vi "Controller 2 Functions.vi"(8 "AutoArmIn":u8, 10 "Controller in":string, 11 "Enabled?":enum16{"Disabled", "Enabled"}(ring)) -> (0 "AutoArm Out":u8)   [LabVIEW 2012, in "BlockParty4150.lvrbt"]
uses:
  BlockParty4150.lvrbt
  <vilib>/NXT/Hardware/Plugins/Tetrix DC Motor/TetrixDCMotorAddress.ctl
  <vilib>/NXT/Hardware/Plugins/Tetrix 180 deg Servo/Tetrix180ServoAddress.ctl
  <vilib>/FTC/FTC Calculate Drive Power - Tank.vi
  <vilib>/NXT/NXTIO Xnodes/NXTIONodeSubVIs/TETRIX IO Move DC Motors.vi
  <vilib>/NXT/NXTIO Xnodes/NXTIONodeSubVIs/TETRIX IO Move Servos.vi
  <vilib>/NXT/NXTIO Xnodes/AddressXNode/NXTIOAddress.xnode
  <vilib>/NXT/Subs/LVHSConnector.ctl
  <vilib>/NXT/NXTIO Xnodes/NXTIOXNode/NXTIO.xnode
  <vilib>/NXT/LegoClasses/BrickReference/BrickReference.lvclass
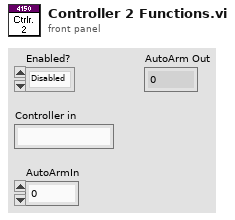
[diagram p1: front panel]
types:
  T1 = typedef "TetrixDCMotorAddress.ctl" = i32
  T2 = cluster{"TetrixDCMotor":T1, "TetrixDCMotor 2":T1}
  T3 = typedef "FTC ControllerState.ctl" = cluster{"Left X":i8, "Left Y":i8, "Right X":i8, "Right Y":i8, "Button Encoding 9-12":u8, "Button Encoding 1-8":u8, "POV":T4}
  T4 = typedef "FTC POVState.ctl" = i8
  T5 = typedef "FTC ButtonState.ctl" = cluster{"Button 1":bool, "Button 2":bool, "Button 3":bool, "Button 4":bool, "Button 5":bool, "Button 6":bool, "Button 7":bool, "Button 8":bool, "Button 9":bool, "Button 10":bool, "Button 11":bool, "Button 12":bool, "POV":T4}
  T6 = typedef "Tetrix180ServoAddress.ctl" = i32
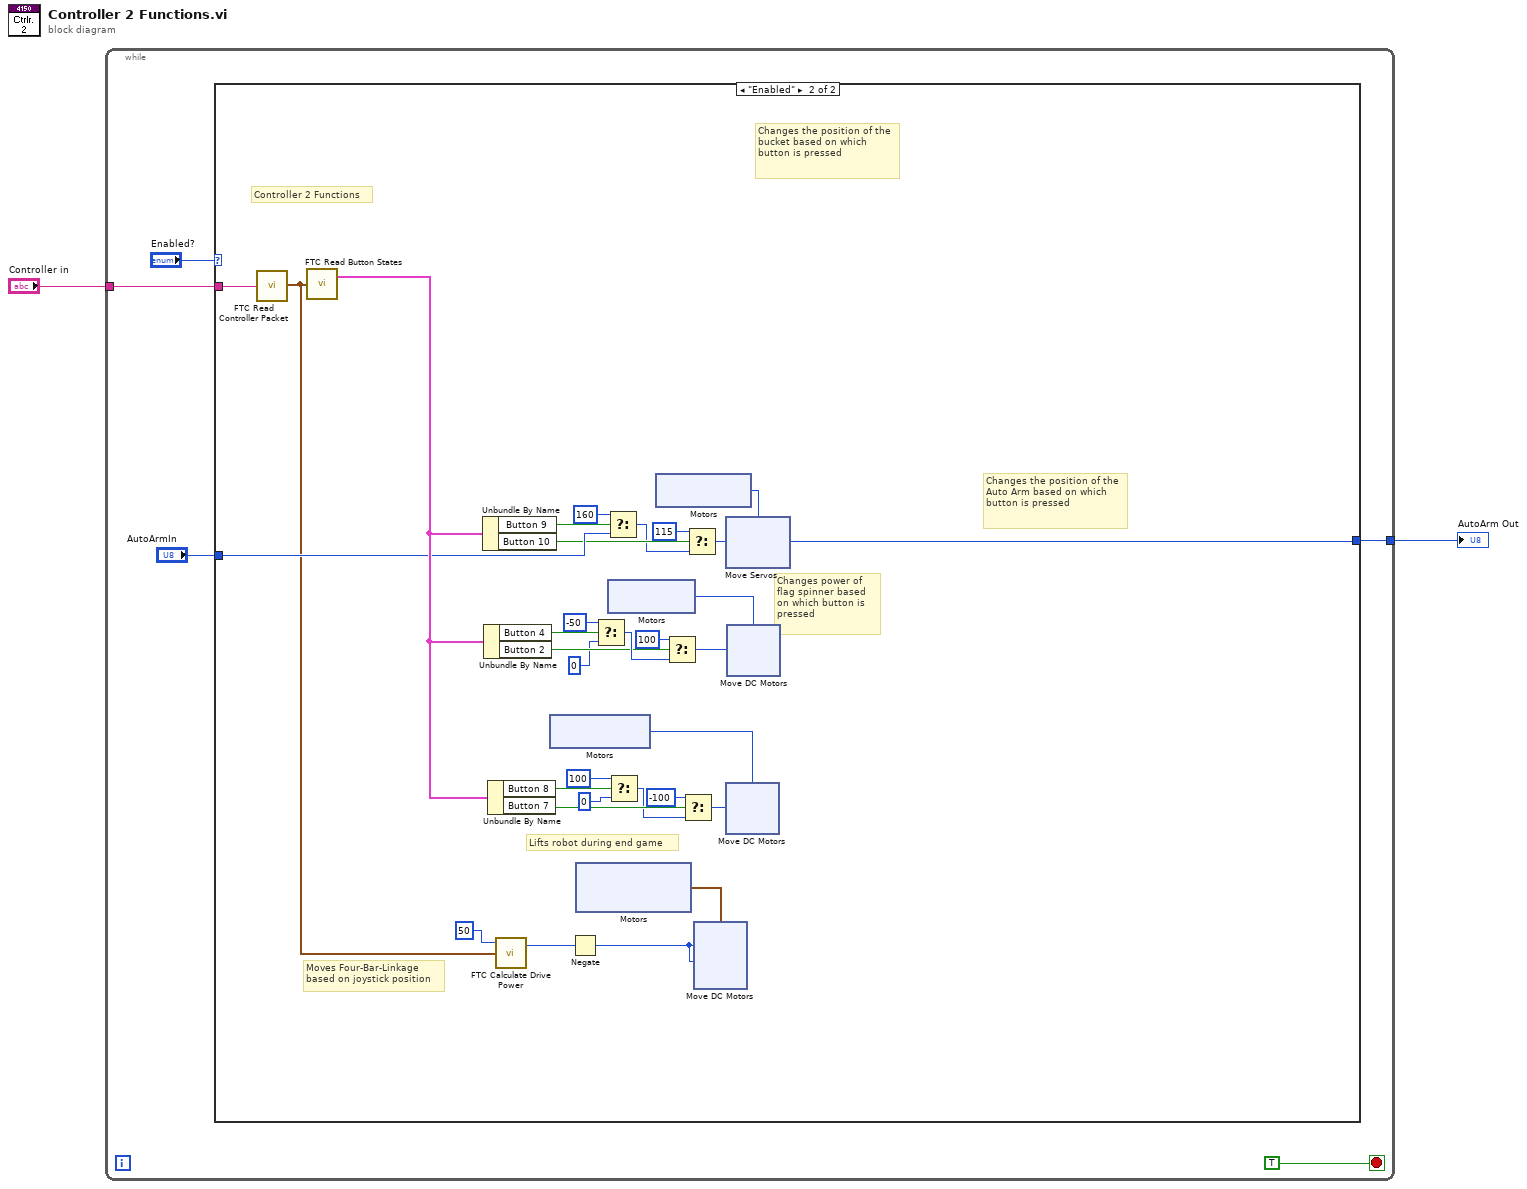
[diagram p0: block diagram]
diagram:
  n1 = while {
    tunnel: [w6] -> w2
    tunnel: "Controller in" -> [w4]
    stop <- TRUE stop-if-true
    n2 = case shown="\"Enabled\"" "Enabled?" {
      tunnel: w4 -> [_ w39]
      tunnel: "AutoArmIn" -> [w8 w37]
      tunnel: [w8 w36] -> w6
      frame "Disabled", Default {
      }
      frame "Enabled" {
        # "Changes the position of the bucket based on which button is pressed"
        # "Changes the position of the Auto Arm based on which button is pressed"
        # "Lifts robot during end game"
        # "Moves Four-Bar-Linkage\nbased on joystick position"
        # "Changes power of\nflag spinner based\non which button is \npressed"
        # "Controller 2 Functions"
        n3 = call <vilib>:"FTC Read Controller Packet.vi"("Packet"=w39) -> ("Controller State"=w12:T3)  [unwired: 4 in]
        n4 = call <vilib>:"FTC Read Button States.vi"("Controller State"=w12) -> ("Button States"=w38:T5)  [unwired: 2 in, 1 out]
        n5 = Unbundle By Name(w38) -> ("Button 9"=w32:bool, "Button 10"=w31:bool)
        n6 = Unbundle By Name(w38) -> ("Button 4"=w27:bool, "Button 2"=w26:bool)
        n7 = Unbundle By Name(w38) -> ("Button 8"=w21:bool, "Button 7"=w16:bool)
        n8 = call-poly <vilib>:"FTC Calculate Drive Power.vi"("Controller State"=w12, "Power Level (50)"=i8 50) -> ("Left Motor Power"=w10:i8)  [unwired: 2 in, 1 out]
        n9 = xnode "Motors"() -> ("Motor"=w20:T1)
        n10 = Negate(x=w10) -> (-x=w9:i8)
        n11 = xnode "Motors"() -> ("Motor"=w35:cluster{"TetrixDCMotor":T1, "TetrixDCMotor":T1})
        n12 = Select(t=i8 -50 ("Position 1"), s=w27, f=i8 0) -> (s? t:f=w28:i8)
        n13 = Select(t=u8 160 ("Position 1"), s=w32, f=w37) -> (s? t:f=w29:u8)
        n14 = xnode "Motors"() -> ("Motor"=w13:T1)
        n15 = Select(t=i8 100, s=w21, f=i8 0 ("Power/Speed 1")) -> (s? t:f=w15:i8)
        n16 = xnode "Motors"() -> ("Motor"=w34:T6)
        n17 = Select(t=i8 100, s=w26, f=w28) -> (s? t:f=w22:i8)
        n18 = Select(t=i8 -100, s=w16, f=w15) -> (s? t:f=w14:i8)
        n19 = Select(t=u8 115 ("f"), s=w31, f=w29) -> (s? t:f=w36:u8)
        n20 = xnode "Move DC Motors"("Power/Speed 2"=w9, "Power/Speed 1"=w9, "Motors"=w35) -> ()  [unwired: 1 in, 1 out]
        n21 = xnode "Move Servos"("Position 1"=w36, "Motors"=w34) -> ()  [unwired: 1 in, 1 out]
        n22 = xnode "Move DC Motors"("Power/Speed 1"=w14, "Motors"=w20) -> ()  [unwired: 1 in, 1 out]
        n23 = xnode "Move DC Motors"("Power/Speed 1"=w22, "Motors"=w13) -> ()  [unwired: 1 in, 1 out]
      }
    }
  }
  "AutoArm Out" <- w2
